vi "Set Amplitude.vi"(8 "error in (no error)":errorcluster, 10 "Output amplitude":dbl=1.0 min=-1.0 max=1.0 format="%#_8pV", 11 "Lock-in in":refnum<class "Lock-in.lvclass">) -> (0 "error out":errorcluster, 3 "Lock-in out":refnum<class "Lock-in.lvclass">)   [LabVIEW 2021, in "Lock-in.lvclass"]
uses:
  Lock-in.lvclass
  Read Lock-in driver.vi
  Write Lock-in driver.vi
  NHMFL_Core/Libraries/Instruments/Instrument Driver/Lock-in Driver/Lock-in Driver.lvclass
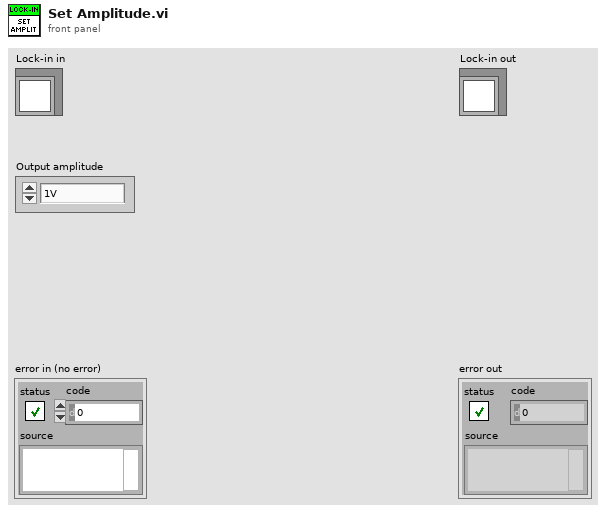
[diagram p1: front panel]
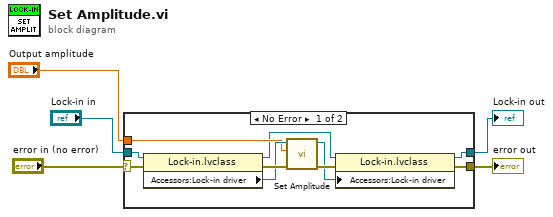
[diagram p0: block diagram]
diagram:
  n1 = case shown="No Error" "error in (no error)" {
    selector: "error in (no error)" -> [w6 w17]
    tunnel: [w7 w17] -> w4
    tunnel: [w11 w16] -> w2
    tunnel: "Lock-in in" -> [w10 w16]
    tunnel: "Output amplitude" -> [w13 _]
    frame No Error {
      n2 = property class="Lock-in.lvclass"(reference=w10, error in=w6) -> (reference out=w12:refnum<class "Lock-in.lvclass">, error out=w15:errorcluster, "Accessors:Lock-in driver"=w14:refnum<class "Lock-in Driver.lvclass">)
      n3 = call-dynamic "Set Amplitude.vi"("error in (no error)"=w15, "Output amplitude"=w13, "Lock-in Driver in"=w14) -> ("error out"=w9:errorcluster, "Lock-in Driver out"=w8:refnum<class "Lock-in Driver.lvclass">)  [unwired: 7 in]
      n4 = property class="Lock-in.lvclass"(reference=w12, error in=w9, "Accessors:Lock-in driver"=w8) -> (reference out=w11:refnum<class "Lock-in.lvclass">, error out=w7:errorcluster)
    }
    frame Error {
    }
  }
  "error out" <- w4
  "Lock-in out" <- w2
